vi "Visualize Map.vi"(11 "map in":refnum<data-value>) -> (3 "map out":refnum<data-value>)   [LabVIEW 2020, in "DS Square.lvlib"]
uses:
  DS Square.lvlib
  Map.ctl
  Square Status.ctl
  Square State.ctl
  Center of Mass.ctl
panel:
  out "Battlefield":i32[][](graph)
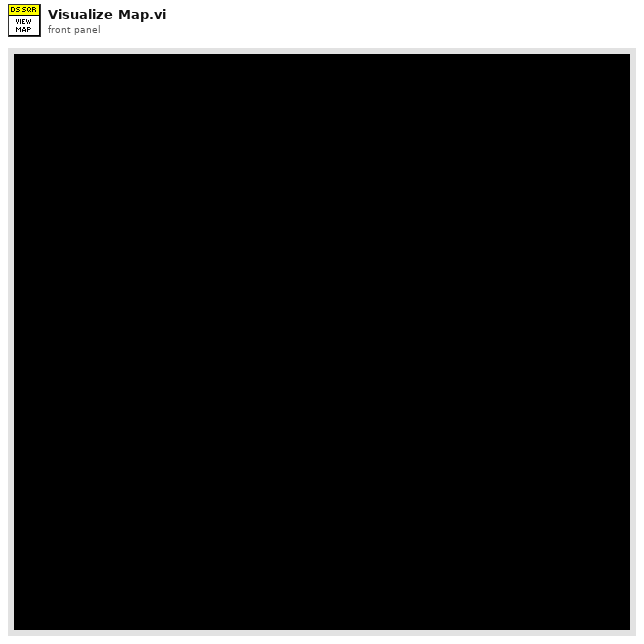
[diagram p1: front panel]
types:
  T1 = typedef "DS Square.lvlib/Square State.ctl" = enum16{"Unknown", "Empty", "Occupied - Active", "Occupied - Cool Down", "Attacked", "Enemy", "Enemy Wall"}
  T2 = typedef "DS Square.lvlib/Map.ctl" = cluster{"squares":T3[][], "center of mass":T4}
  T3 = typedef "DS Square.lvlib/Square Status.ctl" = cluster{"square state":T1, "probability":dbl, "last update":i32}
  T4 = typedef "DS Square.lvlib/Center of Mass.ctl" = cluster{"row":dbl, "col":dbl, "mass":dbl}
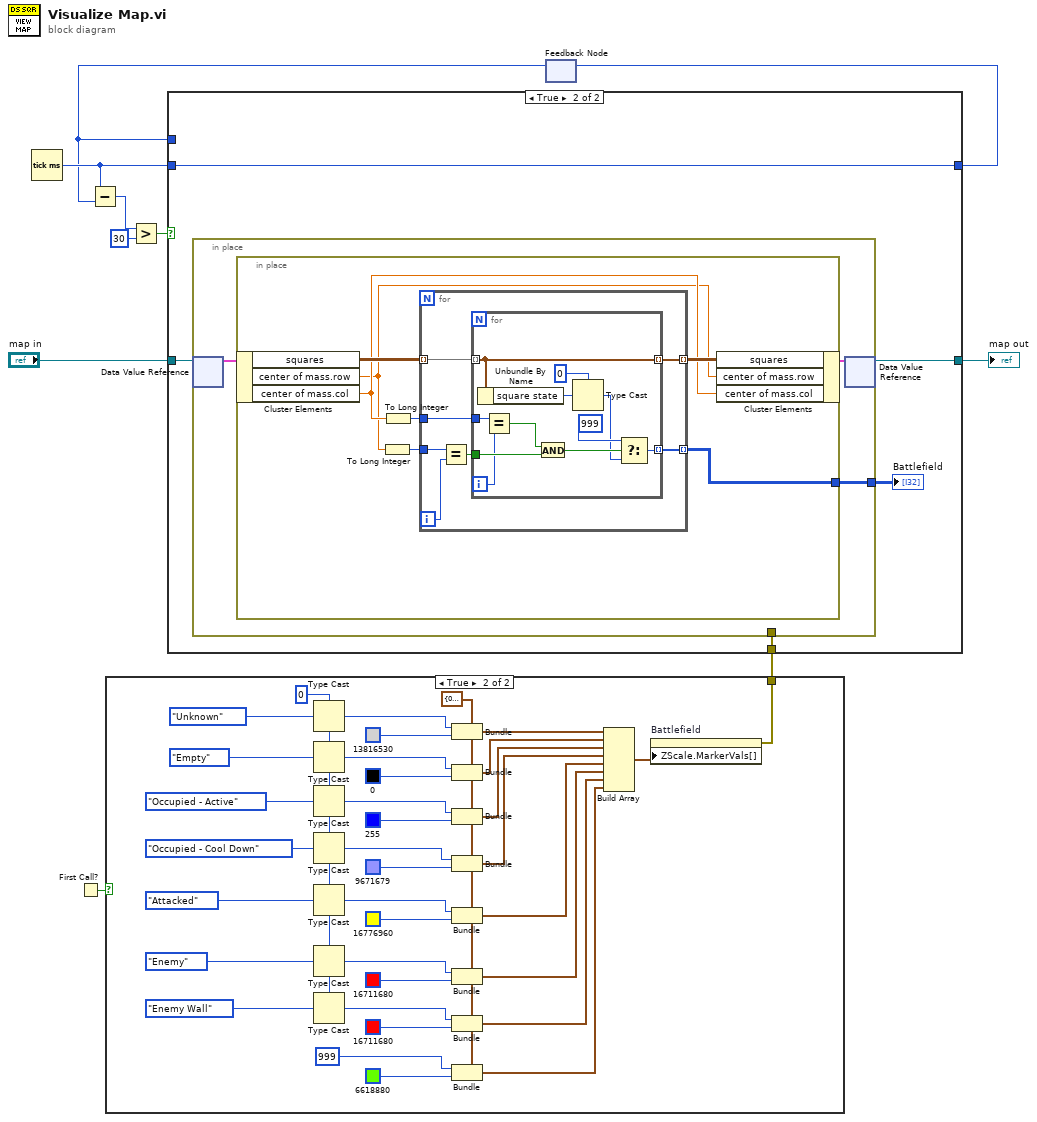
[diagram p0: block diagram]
diagram:
  n1 = Tick Count (ms)() -> (millisecond timer value=w2:u32)
  n2 = First Call?() -> (First Call?: T/F=w4:bool)
  n3 = case shown="True" w4 {
    tunnel: [_ w45] -> w8
    frame False {
    }
    frame True {
      w19 = 0 ("y")
      w28 = cluster{dbl, u32} {0.0, 0}
      n4 = Type Cast(type=w19, x=Square_State."Unknown" ("square state")) -> (*(type *) &x=w24:i32)
      n5 = Type Cast(type=w19, x=Square_State."Empty" ("square state")) -> (*(type *) &x=w20:i32)
      n6 = Type Cast(type=w19, x=Square_State."Occupied - Active" ("square state")) -> (*(type *) &x=w15:i32)
      n7 = Type Cast(type=w19, x=Square_State."Occupied - Cool Down" ("square state")) -> (*(type *) &x=w14:i32)
      n8 = Type Cast(type=w19, x=Square_State."Attacked" ("square state")) -> (*(type *) &x=w13:i32)
      n9 = Type Cast(type=w19, x=Square_State."Enemy" ("square state")) -> (*(type *) &x=w12:i32)
      n10 = Type Cast(type=w19, x=Square_State."Enemy Wall" ("square state")) -> (*(type *) &x=w11:i32)
      n11 = Bundle(cluster=w28, w24, u32 13816530) -> (w41:cluster{dbl, u32})
      n12 = Bundle(cluster=w28, w20, u32 0) -> (w40:cluster{dbl, u32})
      n13 = Bundle(cluster=w28, w15, u32 255) -> (w38:cluster{dbl, u32})
      n14 = Bundle(cluster=w28, w14, u32 9671679) -> (w33:cluster{dbl, u32})
      n15 = Bundle(cluster=w28, w13, u32 16776960) -> (w32:cluster{dbl, u32})
      n16 = Bundle(cluster=w28, w12, u32 16711680) -> (w31:cluster{dbl, u32})
      n17 = Bundle(cluster=w28, w11, u32 16711680) -> (w30:cluster{dbl, u32})
      n18 = Bundle(cluster=w28, 999, u32 6618880) -> (w26:cluster{dbl, u32})
      n19 = Build Array(w41, w40, w38, w33, w32, w31, w30, w26) -> (w44:cluster{dbl, u32}[])
      n20 = property on="Battlefield" class="IntGraph (strict)"("ZScale.MarkerVals[]"=w44) -> (error out=w45:errorcluster)  [unwired: 2 in, 1 out]
    }
  }
  n21 = feedback #1() -> (w1:u32)  [unwired: 1 in]
  n22 = Subtract(x=w2, y=w1) -> (x-y=w7:u32)
  n23 = Greater?(x=w7, y=u32 30) -> (0:w5:bool)
  n24 = case shown="True" w5 {
    tunnel: "map in" -> [w47 w52]
    tunnel: [w47 w51] -> w9
    tunnel: w8 -> [_ w50]
    tunnel: [w46 w48] -> w3
    tunnel: w2 -> [_ w48]
    tunnel: w1 -> [w46 _]
    frame False {
    }
    frame True {
      n25 = in-place {
        in-place-border: w50 -> [_]
        in-place-border: [w53] -> w49
        n26 = in-place-dvr #2(w52) -> (w55:T2)  [unwired: 1 out]
        n27 = in-place {
          in-place-border: [w60] -> w53
          n28 = in-place-cluster #3(w55) -> ("squares"=w62:T3[][], "center of mass.row"=w56:dbl, "center of mass.col"=w57:dbl)
          n29 = To Long Integer(number=w56) -> (32bit integer=w58:i32)
          n30 = To Long Integer(number=w57) -> (32bit integer=w59:i32)
          n31 = for {
            tunnel: w62 -> [w69] mode=indexing
            tunnel: [w68] -> w61 mode=indexing
            tunnel: [w67] -> w60 mode=indexing
            tunnel: w59 -> [w66]
            tunnel: w58 -> [w65]
            i -> [w64]
            n32 = Equal?(x=w65, y=w64) -> (x = y?=w63:bool)
            n33 = for {
              tunnel: w69 -> [w80] mode=indexing
              tunnel: [w80] -> w68 mode=indexing
              tunnel: [w75] -> w67 mode=indexing
              tunnel: w66 -> [w79]
              tunnel: w63 -> [w71]
              i -> [w70]
              n34 = Unbundle By Name(w80) -> ("square state"=w73:T1)
              n35 = Equal?(x=w79, y=w70) -> (x = y?=w78:bool)
              n36 = And(x=w78, y=w71) -> (x .and. y?=w77:bool)
              n37 = Type Cast(type=0 ("y"), x=w73) -> (*(type *) &x=w72:i32)
              n38 = Select(t=999, s=w77, f=w72) -> (s? t:f=w75:i32)
            }
          }
          n39 = in-place-cluster #3("squares"=w61, "center of mass.row"=w56, "center of mass.col"=w57) -> (w54:T2)
        }
        n40 = in-place-dvr #2(w54) -> (w51:refnum<data-value>)  [unwired: 1 out]
      }
      "Battlefield" <- w49
    }
  }
  "map out" <- w9
  n41 = feedback-in #1(w3) -> ()
